vi "Var_SetMultReportingParameters.vi"(8 "error in":errorcluster, 10 "reporting parameters":T1[](array[typedef]), 11 "reporting params in":variant) -> (0 "error out":errorcluster, 2 "replaced?":bool[](array[boolean]), 3 "reporting params out":variant)   [LabVIEW 2013, in "CLM_ErrorHandler.lvlib" / "ErrorReporter.lvclass"]
uses:
  ErrorReporter.lvclass
  ReportingParameter.ctl
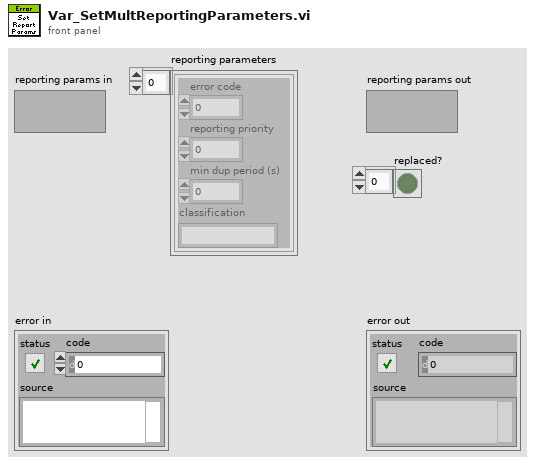
[diagram p1: front panel]
types:
  T1 = typedef "CLM_ErrorHandler.lvlib/ErrorReporter.lvclass/ReportingParameter.ctl" = cluster{"error code":i32, "reporting priority":i32, "min dup period (s)":dbl, "classification":string}
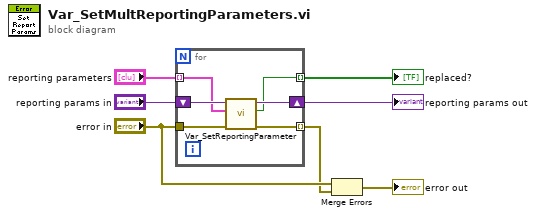
[diagram p0: block diagram]
diagram:
  n1 = for {
    tunnel: "error in" -> [w12]
    tunnel: [w10] -> w2 mode=indexing
    shift-right: [w11] -> w6
    shift-left: "reporting params in" -> [w13]
    tunnel: "reporting parameters" -> [w9] mode=indexing
    tunnel: [w8] -> w4 mode=indexing
    n2 = call "Var_SetReportingParameter.vi"("error in"=w12, "reporting parameter"=w9, "reporting params in"=w13) -> ("error out"=w10:errorcluster, "replaced?"=w8:bool, "reporting params out"=w11:variant)  [unwired: 6 in]
  }
  "reporting params out" <- w6
  "replaced?" <- w4
  n3 = Merge Errors("error in", w2) -> (→"error out":errorcluster)
